vi "Command Drive Distance Delay.vi"(8 "Turn_Distance":dbl=42.0, 9 "Heading":dbl=50.0, 10 "Distance":dbl=42.0, 11 "Startup":bool) -> (0 "Right Wheel":dbl, 1 "Reinit":bool, 2 "Left Wheel":dbl, 3 "Completed":bool=TRUE)   [LabVIEW 2017]
uses:
  Utility VIs/Refnum Names.vi
  Drive/Drive Globals.vi
panel:
  out "Initial Heading":dbl
  in  "Turn Gain":dbl=0.06
  in  "Gain":dbl=0.028
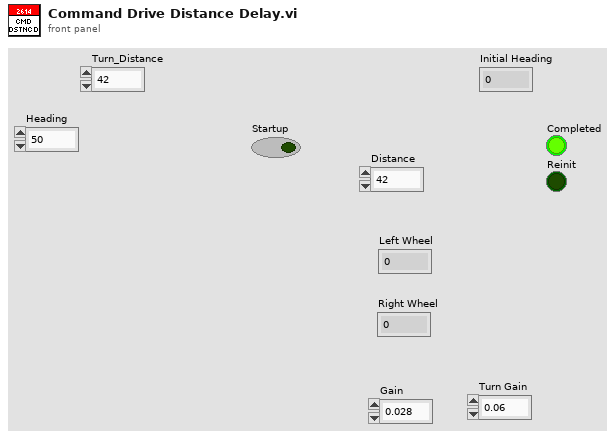
[diagram p1: front panel]
types:
  T1 = typedef "WPI_MotorControlDeviceRef.ctl" = cluster{"DeviceStatus":errorcluster, "Type":T2, "PWM":cluster{"PWM Channel":T3, "DeadBand":T4}, "CAN":cluster{"Device Number":u8, "SetOutput VI Ref":variant, "GetOutput VI Ref":variant, "Enable VI Ref":variant, "Disable VI Ref":variant, "Data":variant}, "Invert":bool, "DIO PWM":cluster{"PWM \"Enable\" Channel":T3, "DIOChannel":T5, "PWM Rate":dbl}}
  T2 = typedef "WPI_MotorControlType.ctl" = enum16{"PWM", "CAN", "DIO PWM"}
  T3 = typedef "FPGA_DIOPWMChannel.ctl" = enum8{"PWM 0", "PWM 1", "PWM 2", "PWM 3", "PWM 4", "PWM 5", "PWM 6", "PWM 7", "PWM 8", "PWM 9", "PWM MXP 0", "PWM MXP 1", "PWM MXP 2", "PWM MXP 3", "PWM MXP 4", "PWM MXP 5", "PWM MXP 6", "PWM MXP 7", "PWM MXP 8", "PWM MXP 9", "Invalid"}
  T4 = typedef "WPI_PWMDeadband.ctl" = cluster{"Name":string, "maxPositivePwm":i32, "minPositivePwm":i32, "centerPwm":i32, "maxNegativePwm":i32, "minNegativePwm":i32, "angularRange":u16}
  T5 = typedef "FPGA_DIOChannel.ctl" = enum8{"DIO 0", "DIO 1", "DIO 2", "DIO 3", "DIO 4", "DIO 5", "DIO 6", "DIO 7", "DIO 8", "DIO 9", "DIO MXP 0", "DIO MXP 1", "DIO MXP 2", "DIO MXP 3", "DIO MXP 4", "DIO MXP 5", "DIO MXP 6", "DIO MXP 7", "DIO MXP 8", "DIO MXP 9", "DIO MXP 10", "DIO MXP 11", "DIO MXP 12", "DIO MXP 13", "DIO MXP 14", "DIO MXP 15", "SPI Port CS1", "SPI Port CS2", "SPI Port CS3", "SPI Port MISO", "SPI Port MOSI", "Invalid"}
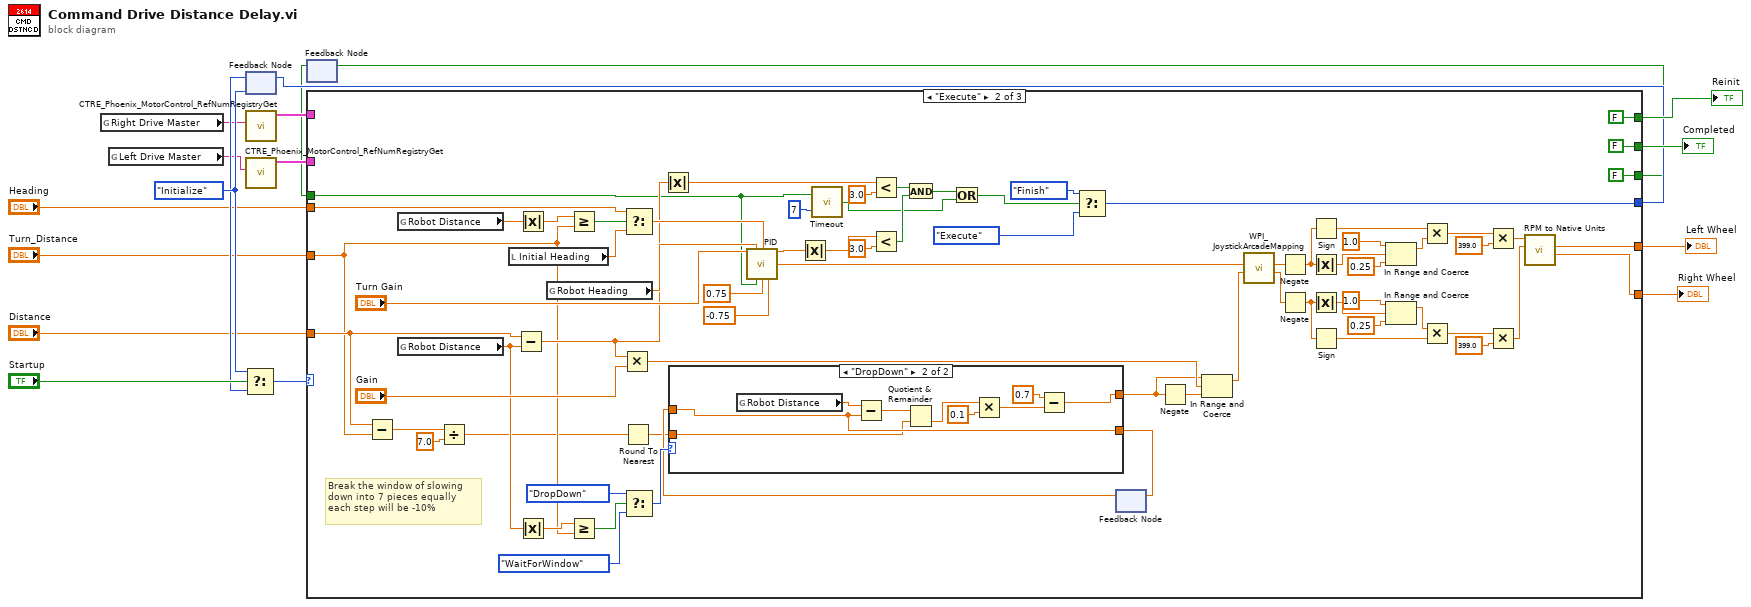
[diagram p0: block diagram]
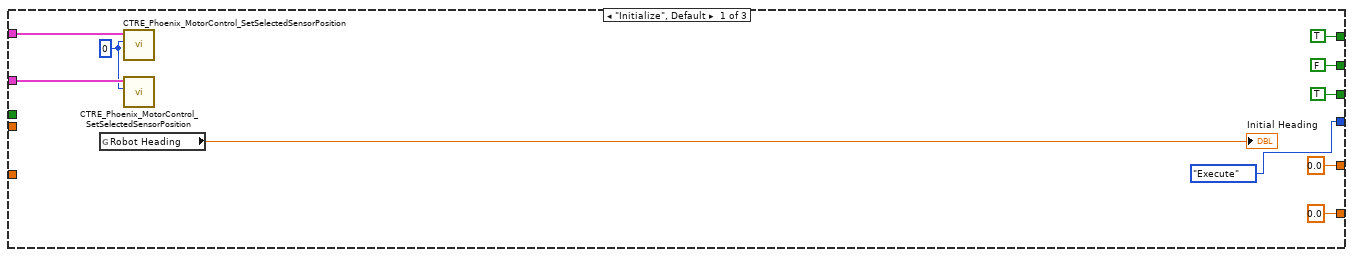
[diagram p2: hidden frame]
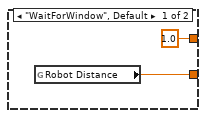
[diagram p3: hidden frame]
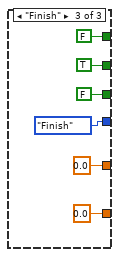
[diagram p4: hidden frame]
diagram:
  w16 = enum16{"Initialize", "Execute", "Finish"}."Initialize"
  n1 = global read "Refnum Names.vi" "Right Drive Master"() -> (w7:string)
  n2 = global read "Refnum Names.vi" "Left Drive Master"() -> (w8:string)
  n3 = feedback #1(w16) -> (w12:enum16{"Initialize", "Execute", "Finish"})
  n4 = Select(t=w16, s="Startup", f=w12) -> (s? t:f=w17:enum16{"Initialize", "Execute", "Finish"})
  n5 = call <vilib>:"CTRE_Phoenix_MotorControl_RefNumRegistryGet.vi"("refnum name"=w7) -> ("PhoenixMotorControlDevRef"=w6:T1)  [unwired: 9 in, 1 out]
  n6 = call <vilib>:"CTRE_Phoenix_MotorControl_RefNumRegistryGet.vi"("refnum name"=w8) -> ("PhoenixMotorControlDevRef"=w5:T1)  [unwired: 9 in, 1 out]
  n7 = feedback #2() -> (w2:bool)  [unwired: 1 in]
  n8 = case shown="\"Execute\"" w17 {
    tunnel: [FALSE FALSE TRUE] -> w15
    tunnel: [TRUE FALSE FALSE] -> w14
    tunnel: [enum16{"Initialize", "Execute", "Finish"}."Execute" w96 enum16{"Initialize", "Execute", "Finish"}."Finish"] -> w13
    tunnel: "Distance" -> [_ w35 _]
    tunnel: [0.0 ("Left Wheel Velocity") w55 0.0] -> w10
    tunnel: [0.0 ("Right Wheel Velocity") w54 0.0] -> w9
    tunnel: w6 -> [w22 _ _]
    tunnel: w5 -> [w23 _ _]
    tunnel: "Heading" -> [_ w51 _]
    tunnel: [TRUE FALSE FALSE] -> w3
    tunnel: w2 -> [_ w29 _]
    tunnel: "Turn_Distance" -> [_ w34 _]
    frame "Initialize", Default {
      w21 = 0
      n9 = global read "Drive Globals.vi" "Robot Heading"() -> (→"Initial Heading":dbl)
      n10 = call <vilib>:"CTRE_Phoenix_MotorControl_SetSelectedSensorPosition.vi"("New Sensor Position"=w21, "PhoenixMotorControlDevRef"=w22) -> ()  [unwired: 8 in, 2 out]
      n11 = call <vilib>:"CTRE_Phoenix_MotorControl_SetSelectedSensorPosition.vi"("New Sensor Position"=w21, "PhoenixMotorControlDevRef"=w23) -> ()  [unwired: 8 in, 2 out]
    }
    frame "Execute" {
      # "Break the window of slowing\ndown into 7 pieces equally\neach step will be -10%"
      n12 = Subtract(x=w35, y=w34) -> (x-y=w33:dbl)
      n13 = global read "Drive Globals.vi" "Robot Distance"() -> (w48:dbl)
      n14 = global read "Drive Globals.vi" "Robot Distance"() -> (w44:dbl)
      n15 = Divide(x=w33, y=7.0) -> (x/y=w31:dbl)
      n16 = local read "Initial Heading"() -> (w50:dbl)
      n17 = Subtract(x=w35, y=w44) -> (x-y=w38:dbl)
      n18 = Absolute Value(x=w48) -> (abs(x)=w47:dbl)
      n19 = Absolute Value(x=w44) -> (abs(x)=w46:dbl)
      n20 = global read "Drive Globals.vi" "Robot Heading"() -> (w92:dbl)
      n21 = Greater Or Equal?(x=w47, y=w34) -> (x >= y?=w49:bool)
      n22 = Greater Or Equal?(x=w46, y=w34) -> (x >= y?=w40:bool)
      n23 = Multiply(x=w38, y="Gain") -> (x*y=w90:dbl)
      n24 = Round To Nearest(number=w31) -> (nearest integer value=w30:dbl)
      n25 = Select(t=w51, s=w49, f=w50) -> (s? t:f=w52:dbl)
      n26 = Select(t=enum16{"WaitForWindow", "DropDown"}."DropDown" ("Ramp Down"), s=w40, f=enum16{"WaitForWindow", "DropDown"}."WaitForWindow" ("Ramp Down")) -> (s? t:f=w43:enum16{"WaitForWindow", "DropDown"})
      n27 = Absolute Value(x=w38) -> (abs(x)=w94:dbl)
      n28 = call "PID.vi"("Kp"="Turn Gain", "Process Variable"=w92, "Goal"=w52, "Reinit"=w29, "Max Ouput"=0.75, "Min Output"=-0.75) -> ("Current Error"=w81:dbl, "Command"=w80:dbl)  [unwired: 7 in, 1 out]
      n29 = Absolute Value(x=w81) -> (abs(x)=w83:dbl)
      n30 = call "Timeout.vi"("Timeout"=u32 7, "Initialize"=w29) -> ("Timed Out?"=w72:bool)
      n31 = Less?(x=w94, y=3.0) -> (x < y?=w85:bool)
      n32 = Less?(x=w83, y=3.0) -> (x < y?=w82:bool)
      n33 = And(x=w85, y=w82) -> (x .and. y?=w86:bool)
      n34 = Or(x=w86, y=w72) -> (x .or. y?=w73:bool)
      n35 = Select(t=enum16{"Initialize", "Execute", "Finish"}."Finish", s=w73, f=enum16{"Initialize", "Execute", "Finish"}."Execute") -> (s? t:f=w96:enum16{"Initialize", "Execute", "Finish"})
      n36 = feedback #3() -> (w37:dbl)  [unwired: 1 in]
      n37 = case shown="\"DropDown\"" w43 {
        tunnel: [1.0 w103] -> w39
        tunnel: w37 -> [_ w109]
        tunnel: [w100 w109] -> w36
        tunnel: w30 -> [_ w102]
        frame "WaitForWindow", Default {
          n38 = global read "Drive Globals.vi" "Robot Distance"() -> (w100:dbl)
        }
        frame "DropDown" {
          n39 = global read "Drive Globals.vi" "Robot Distance"() -> (w110:dbl)
          n40 = Subtract(x=w110, y=w109) -> (x-y=w108:dbl)
          n41 = Quotient & Remainder(x=w108, y=w102) -> (floor(x/y)=w106:dbl)  [unwired: 1 out]
          n42 = Multiply(x=w106, y=0.1) -> (x*y=w105:dbl)
          n43 = Subtract(x=0.7, y=w105) -> (x-y=w103:dbl)
        }
      }
      n44 = feedback-in #3(w36) -> ()
      n45 = Negate(x=w39) -> (-x=w45:dbl)
      n46 = In Range and Coerce(upper limit=w39, x=w90, lower limit=w45) -> (coerced(x)=w79:dbl)  [unwired: 1 out]
      n47 = call <vilib>:"WPI_JoystickArcadeMapping.vi"("Y axis value"=w79, "X axis value"=w80) -> ("Right Motor Value"=w77:dbl, "Left Motor Value"=w78:dbl)  [unwired: 8 in]
      n48 = Negate(x=w78) -> (-x=w68:dbl)
      n49 = Negate(x=w77) -> (-x=w69:dbl)
      n50 = Sign(1:w68) -> (0:w67:dbl)
      n51 = Absolute Value(x=w68) -> (abs(x)=w71:dbl)
      n52 = Absolute Value(x=w69) -> (abs(x)=w70:dbl)
      n53 = Sign(1:w69) -> (0:w62:dbl)
      n54 = In Range and Coerce(upper limit=1.0, x=w71, lower limit=0.25) -> (coerced(x)=w66:dbl)  [unwired: 1 out]
      n55 = In Range and Coerce(upper limit=1.0, x=w70, lower limit=0.25) -> (coerced(x)=w63:dbl)  [unwired: 1 out]
      n56 = Multiply(x=w67, y=w66) -> (x*y=w65:dbl)
      n57 = Multiply(x=w63, y=w62) -> (x*y=w64:dbl)
      n58 = Multiply(x=w65, y=399.0) -> (x*y=w57:dbl)
      n59 = Multiply(x=w64, y=399.0) -> (x*y=w56:dbl)
      n60 = call "RPM to Native Units.vi"("Right RPM"=w56, "Left RPM"=w57) -> ("Right Out"=w54:dbl, "Left Out"=w55:dbl)  [unwired: 6 in, 1 out]
    }
    frame "Finish" {
    }
  }
  "Completed" <- w15
  "Reinit" <- w14
  "Left Wheel" <- w10
  "Right Wheel" <- w9
  n61 = feedback-in #1(w13) -> ()
  n62 = feedback-in #2(w3) -> ()
